vi "Create_New_Build.vi"(6 "buildSpecName":string, 7 "Programmatic? (false)":bool, 8 "error in (no error)":errorcluster, 9 "buildObject":T1, 10 "Destination Path":path, 11 "AB_EXE in":refnum<class "AB_EXE.lvclass">) -> (0 "error out":errorcluster, 3 "AB_EXE out":refnum<class "AB_EXE.lvclass">)   [LabVIEW 2020, in "AB_EXE.lvclass"]
uses:
  <vilib>/AppBuilder/AB_Classes/EXE/AB_EXE.lvclass
  e:/builds/penguin/labview/branches/2020/dev/dist/vi.lib/AppBuilder/AB_Classes/TargetFile/AB_Targetfile.lvclass
  <resource>/Framework/Providers/API/ItemRef.ctl
  <vilib>/AppBuilder/AB_TargetFileType.ctl
  <resource>/Framework/Providers/Common/provcom_StringGlobals.vi
  <vilib>/AppBuilder/AB_Classes/Application/AB_Application.lvclass
  <vilib>/AppBuilder/AB_Classes/TargetFile/AB_Targetfile.lvclass
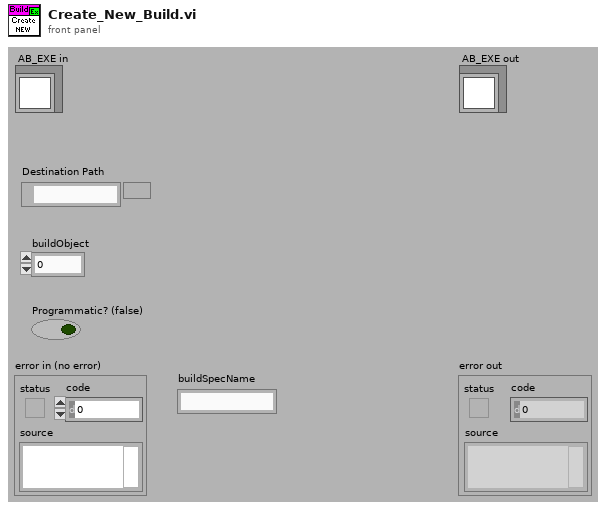
[diagram p1: front panel]
types:
  T1 = typedef "ItemRef.ctl" = u64
  T2 = typedef "AB_TargetFileType.ctl" = enum16{"EXE", "DLL", "RTEXE"}
  T3 = enum32{"invalid OS target", "Mac OS", "Windows 3.1", "Windows 95/NT", "Solaris 1", "Solaris 2", "HP-UX", "PowerMAX", "Linux", "Irix", "Rhapsody", "BeOS", "AIX", "OSF1", "VxWorks", "PharLap", "Carbon", "RTX", "Windows x64", "Linux x64", "Mac OS X x64"}
  T4 = typedef "AB_Targetfile.ctl" = cluster{"targetfileName":string, "targetfileGUID":string, "enableDebugging":bool, "versionInfo":cluster{"productName":string, "legalCopyright":string, "companyName":string, "internalName":string, "fileDescription":string}, "eng_consolidatedTypeInfo":string, "fastFileFormat":bool, "eng_LEIFBuildData":u32, "versionIndependent":bool}
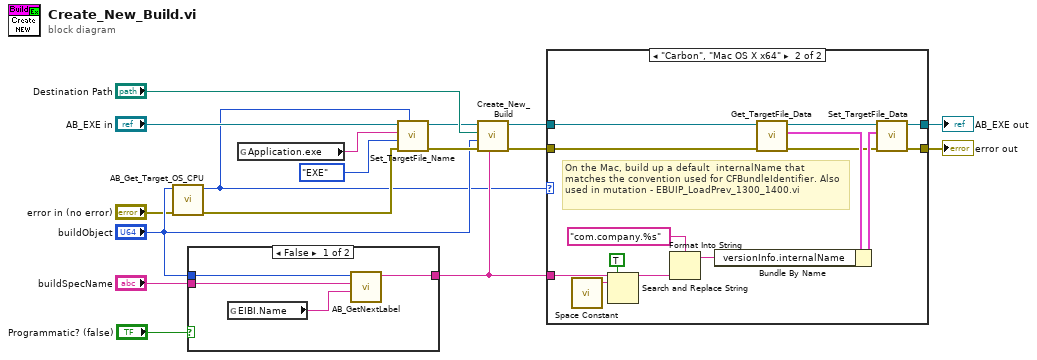
[diagram p0: block diagram]
diagram:
  n1 = call <resource>:"AB_Get_Target_OS_CPU.vi"("error in (no error)"="error in (no error)", "Object"="buildObject") -> ("error out"=w2:errorcluster, "Target Operating System"=w1:T3)  [unwired: 7 in, 1 out]
  n2 = case shown="False" "Programmatic? (false)" {
    tunnel: [w21 w22] -> w9
    tunnel: "buildObject" -> [w20 _]
    tunnel: "buildSpecName" -> [w19 w22]
    frame False {
      n3 = global read "provcom_StringGlobals.vi" "EIBI.Name"() -> (w18:string)
      n4 = call <vilib>:"AB_GetNextLabel.vi"("default name"=w18, "supplied name"=w19, "buildObject"=w20) -> ("New label"=w21:string)  [unwired: 3 in, 5 out]
    }
    frame True {
    }
  }
  n5 = global read "provcom_StringGlobals.vi" "Application.exe"() -> (w13:string)
  n6 = call-dynamic "Set_TargetFile_Name.vi"("Target Operating System"=w1, "error in (no error)"=w2, "Target file type"=AB_TargetFileType."EXE", "Target file name"=w13, "AB_Targetfile in"="AB_EXE in") -> ("error out"=w14:errorcluster, "AB_Targetfile out"=w15:refnum<class "AB_EXE.lvclass">)  [unwired: 5 in]
  n7 = call-parent "Create_New_Build.vi"("buildSpecName"=w9, "error in (no error)"=w14, "buildObject"="buildObject", "Destination Path"="Destination Path", "AB_Application in"=w15) -> ("error out"=w6:errorcluster, "AB_Application out"=w8:refnum<class "AB_EXE.lvclass">)  [unwired: 1 in, 4 out]
  n8 = case shown="\"Carbon\", \"Mac OS X x64\"" w1 {
    tunnel: w9 -> [_ w26]
    tunnel: [w24 w32] -> w7
    tunnel: w8 -> [w24 w33]
    tunnel: w6 -> [w23 w31]
    tunnel: [w23 w30] -> w5
    frame Default {
    }
    frame "Carbon", "Mac OS X x64" {
      # "On the Mac, build up a default  internalName that matches the convention used for CFBundleIdentifier. Also used in mutation - EBUIP_LoadPrev_1300_1400.vi"
      n9 = call <vilib>:"Space Constant.vi"() -> ("String"=w27:string)
      n10 = Search and Replace String(replace all?=TRUE ("replace all? (F)"), input string=w26, search string=w27) -> (result string=w25:string)  [unwired: 5 in, 3 out]
      n11 = Format Into String(format string="com.company.%s", w25) -> (resulting string=w29:string)  [unwired: 2 in, 1 out]
      n12 = call <vilib>:"Get_TargetFile_Data.vi"("error in (no error)"=w31, "AB_Targetfile in"=w33) -> ("error out"=w35:errorcluster, "data"=w36:T4, "AB_Targetfile out"=w34:refnum<class "AB_EXE.lvclass">)  [unwired: 7 in]
      n13 = Bundle By Name(cluster=w36, "versionInfo.internalName"=w29) -> (w37:T4)
      n14 = call <vilib>:"Set_TargetFile_Data.vi"("error in (no error)"=w35, "data"=w37, "AB_Targetfile in"=w34) -> ("error out"=w30:errorcluster, "AB_Targetfile out"=w32:refnum<class "AB_EXE.lvclass">)  [unwired: 7 in]
    }
  }
  "error out" <- w5
  "AB_EXE out" <- w7
